vi "Keithley 24XX Read Multiple - SW Trigger.vi"() -> ()   [LabVIEW 2022 SP3]
doc: "This example shows how to configure a measurement, set up triggering, trigger a measurement, and retrieve a measurement. It shows how to use the low-level Data VIs to retrieve data from the SourceMeter."
uses:
  Keithley 24XX.lvlib
  Initialize Folder/D/Download/Keithley 24XX/Public/Data/Low Level/Fetch (Measurements).vi
panel:
  in  "Source Mode  (0: Voltage)":u16(ring) items=["Voltage", "Current"]
  in  "Timeout (10000 ms)":u32=10000
  out "Waveform Graph":sgl[][](graph)
  in  "Output Level (0)":dbl
  in  "Compliance  Level (0.1)":dbl=0.1
  in  "Serial Configuration":T1={"Baud Rate"=9600, "Parity"=0, "Data Bits"=8, "Stop Bits"=10, "Flow Control"=0} {"Flow Control" items=["None", "XON/XOFF", "RTS/CTS", "XON/XOFF & RTS/CTS", "DTR/DSR", "XON/XOFF & DTR/DSR"]; "Stop Bits" items=["1.0"=10, "1.5"=15, "2.0"=20]; "Data Bits" items=["7"=7, "8"=8]; "Parity" items=["None", "Odd", "Even", "Mark", "Space"]; "Baud Rate" items=["300"=300, "600"=600, "1200"=1200, "2400"=2400, "4800"=4800, "9600"=9600, "19200"=19200]}
  in  "Sample Count (10)":i32=10 format="%#.6g"
  in  "Trigger Count (5)":i32=5 format="%#.6g"
  in  "VISA resource name":refnum<visa-resource-name>
  # "(c) 2006 - 2015 National Instruments.  ALL RIGHTS RESERVED."
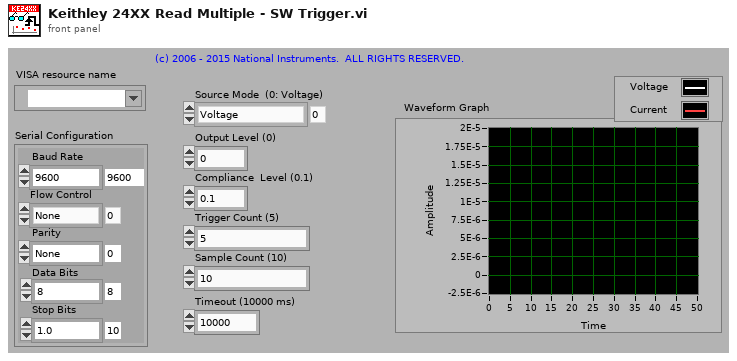
[diagram p1: front panel]
types:
  T1 = cluster{"Baud Rate":u32, "Parity":u16, "Data Bits":u16, "Stop Bits":u16, "Flow Control":u16}
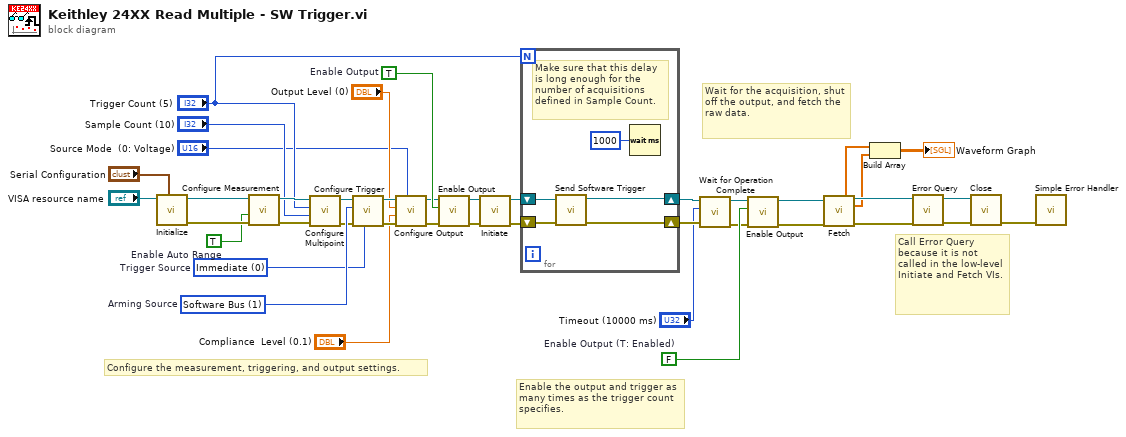
[diagram p0: block diagram]
diagram:
  w21 = FALSE  # Enable Output (T: Enabled)
  w24 = TRUE  # Enable Output
  w27 = u16 1 items=["Immediate", "Software Bus", "Timer", "Manual", "Trigger Link", "Rising SOT Pulse", "Falling SOT Pulse", "Rising or Falling SOT Pulse"]  # Arming Source
  w11 = u16 0 items=["Immediate", "Trigger Link"]  # Trigger Source
  w37 = TRUE  # Enable Auto Range
  # "Wait for the acquisition, shut off the output, and fetch the raw data."
  # "Enable the output and trigger as many times as the trigger count specifies."
  # "Configure the measurement, triggering, and output settings."
  # "Call Error Query because it is not called in the low-level Initiate and Fetch VIs."
  n1 = call "Initialize.vi"("Serial Configuration"="Serial Configuration", "VISA resource name"="VISA resource name") -> ("error out"=w39:errorcluster, "VISA resource name out"=w40:refnum<visa-resource-name>)  [unwired: 8 in]
  n2 = call "Configure Measurement.vi"("error in (no error)"=w39, "Enable Auto Range (T:Enable)"=w37, "VISA resource name"=w40) -> ("error out"=w28:errorcluster, "VISA resource name out"=w29:refnum<visa-resource-name>)  [unwired: 7 in]
  n3 = call "Configure Multipoint.vi"("error in (no error)"=w28, "Trigger Count (1)"="Sample Count (10)", "Number of Times to Arm (1)"="Trigger Count (5)", "VISA resource name"=w29) -> ("error out"=w25:errorcluster, "VISA resource name out"=w26:refnum<visa-resource-name>)  [unwired: 6 in]
  n4 = call "Configure Trigger.vi"("Trigger Source (0: Immediate)"=w11, "error in (no error)"=w25, "Arming Source  (0: Immediate)"=w27, "VISA resource name"=w26) -> ("error out"=w17:errorcluster, "VISA resource name out"=w18:refnum<visa-resource-name>)  [unwired: 6 in]
  n5 = call "Configure Output.vi"("Source Mode  (0: Voltage)"="Source Mode  (0: Voltage)", "error in (no error)"=w17, "Compliance  Level (0.1)"="Compliance  Level (0.1)", "Output Level (0)"="Output Level (0)", "VISA resource name"=w18) -> ("error out"=w15:errorcluster, "VISA resource name out"=w16:refnum<visa-resource-name>)  [unwired: 5 in]
  n6 = call "Enable Output.vi"("error in (no error)"=w15, "Enable Output (T: Enable)"=w24, "VISA resource name"=w16) -> ("error out"=w22:errorcluster, "VISA resource name out"=w23:refnum<visa-resource-name>)  [unwired: 7 in]
  n7 = call "Initiate.vi"("error in (no error)"=w22, "VISA resource name"=w23) -> ("error out"=w36:errorcluster, "VISA resource name out"=w35:refnum<visa-resource-name>)  [unwired: 8 in]
  n8 = for {
    N: "Trigger Count (5)" -> [_]
    shift-right: [w43] -> w7
    shift-left: w36 -> [w44]
    shift-right: [w42] -> w8
    shift-left: w35 -> [w45]
    # "Make sure that this delay is long enough for the number of acquisitions defined in Sample Count."
    n9 = call "Send Software Trigger.vi"("error in (no error)"=w44, "VISA resource name"=w45) -> ("error out"=w43:errorcluster, "VISA resource name out"=w42:refnum<visa-resource-name>)  [unwired: 8 in]
    n10 = Wait (ms)(milliseconds to wait=u32 1000) -> ()  [unwired: 1 out]
  }
  n11 = call "Wait for Operation Complete.vi"("error in (no error)"=w7, "Timeout (10000 ms)"="Timeout (10000 ms)", "VISA resource name"=w8) -> ("error out"=w6:errorcluster, "VISA resource name out"=w5:refnum<visa-resource-name>)  [unwired: 7 in]
  n12 = call "Enable Output.vi"("error in (no error)"=w6, "Enable Output (T: Enable)"=w21, "VISA resource name"=w5) -> ("error out"=w19:errorcluster, "VISA resource name out"=w20:refnum<visa-resource-name>)  [unwired: 7 in]
  n13 = call-poly "Fetch.vi"("VISA resource name"=w20, "error in (no error)"=w19) -> ("Voltage"=w14:sgl[], "VISA resource name out"=w30:refnum<visa-resource-name>, "Current"=w13:sgl[], "error out"=w31:errorcluster)  [unwired: 7 in, 3 out]
  n14 = Build Array(w14, w13) -> (→"Waveform Graph":sgl[][])
  n15 = call "Error Query.vi"("error in (no error)"=w31, "VISA resource name"=w30) -> ("error out"=w32:errorcluster, "VISA resource name out"=w33:refnum<visa-resource-name>)  [unwired: 6 in, 2 out]
  n16 = call "Close.vi"("error in (no error)"=w32, "VISA resource name"=w33) -> ("error out"=w38:errorcluster)  [unwired: 9 in]
  n17 = call <vilib>:"Simple Error Handler.vi"("error in (no error)"=w38) -> ()  [unwired: 4 in, 5 out]
